vi "GEA3 Heat Pump ERD List.vi"(8 "error in (no error)":errorcluster, 11 "Enable Heat Pump List":bool) -> (0 "error out":errorcluster, 2 "Headers":string[](array[string]), 3 "Read ERD List":T1[](array[typedef]) {"ERD Number" format="%.0x"})   [LabVIEW 2020]
uses:
  type defs/ERD Read Data In.ctl
  type defs/Data Type.ctl
  <vilib>/Utility/error.llb/whitespace.ctl
  library/GEA2_Toolkit.lvlib
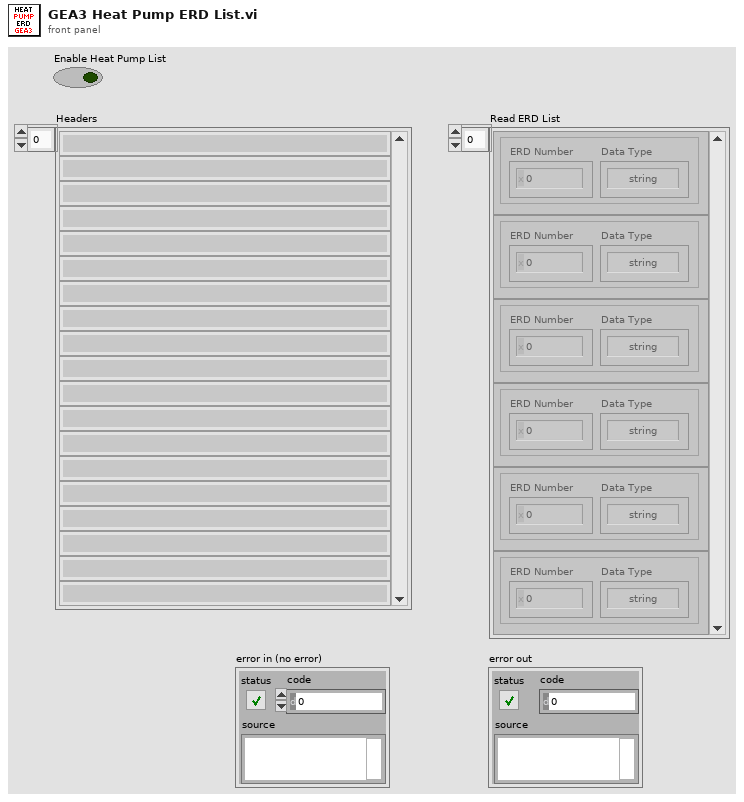
[diagram p1: front panel]
types:
  T1 = typedef "GEA2_Toolkit.lvlib/ERD Read Data In.ctl" = cluster{"ERD Number":u16, "Data Type":T2}
  T2 = typedef "GEA2_Toolkit.lvlib/Data Type.ctl" = enum16{"string", "boolean", "uint8_t", "uint16_t", "uint32_t", "uint64_t", "int8_t", "int16_t", "int32_t", "int64_t"}
  T3 = typedef "whitespace.ctl" = u16
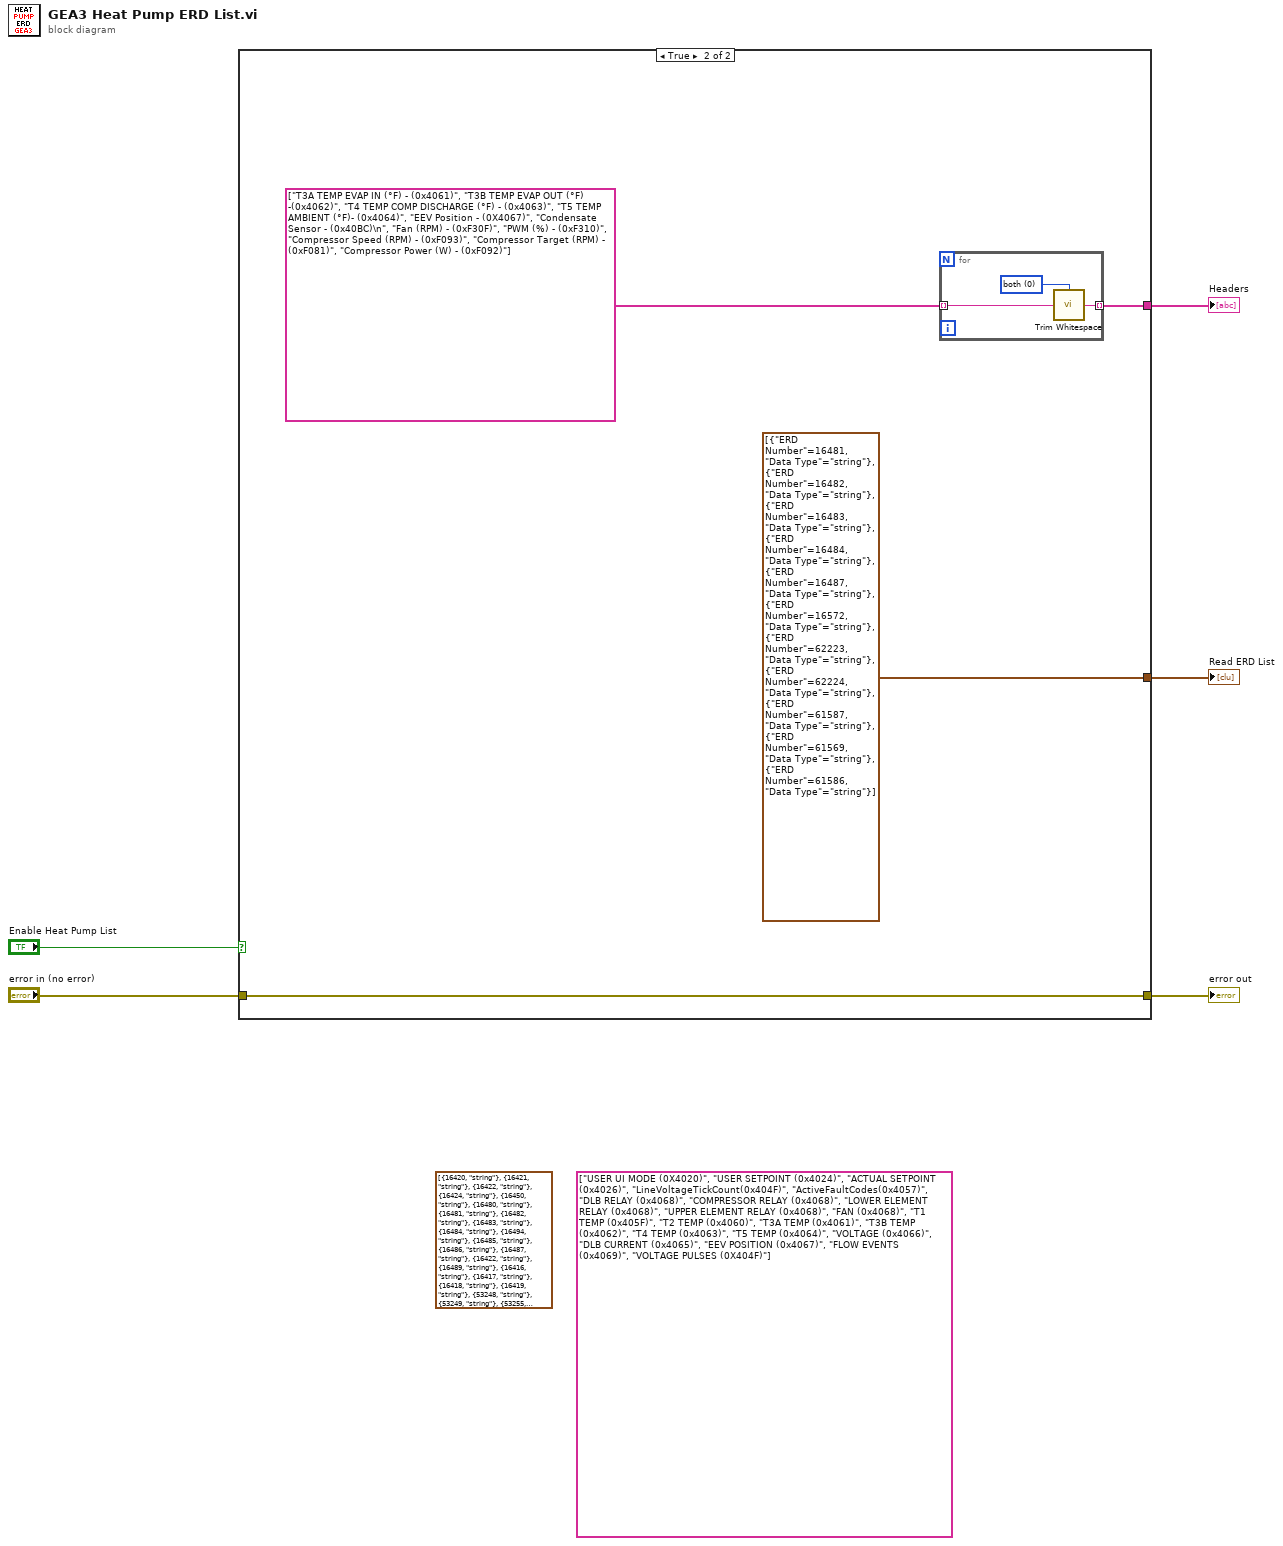
[diagram p0: block diagram]
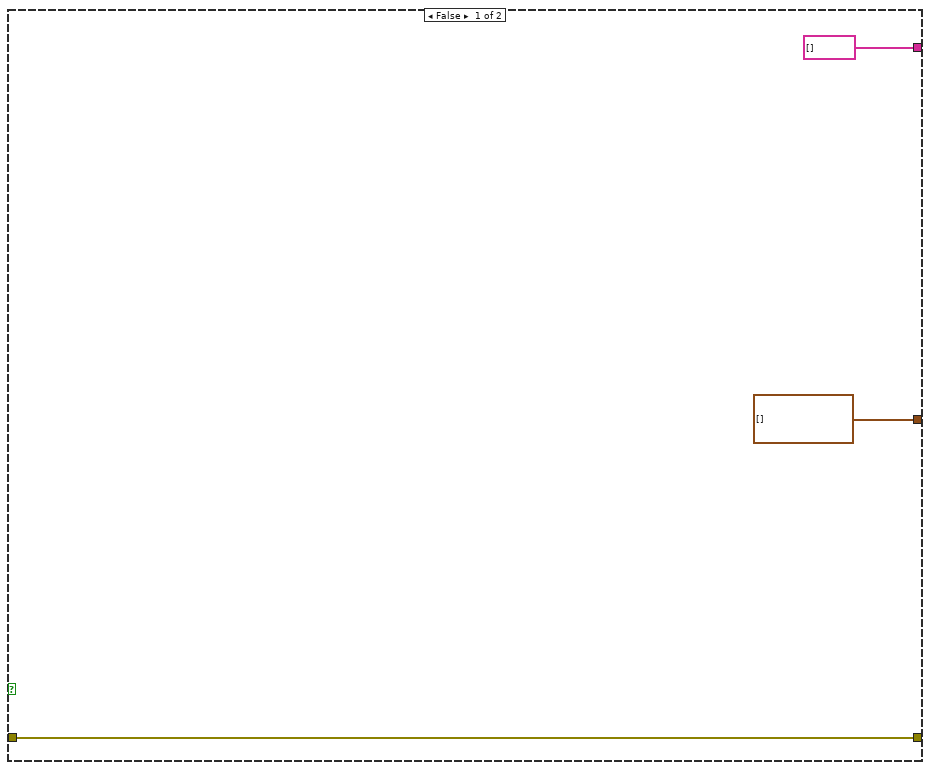
[diagram p2: hidden frame]
diagram:
  (unwired) T1[] [{"ERD Number"=16420, "Data Type"=enum."string"}, {"ERD Number"=16421, "Data Type"=enum."string"}, {"ERD Number"=16422, "Data Type"=enum."string"}, {"ERD Number"=16424, "Data Type"=enum."string"}, {"ERD Number"=16450, "Data Type"=enum."string"}, {"ERD Number"=16480, "Data Type"=enum."string"}, {"ERD Number"=16481, "Data Type"=enum."string"}, {"ERD Number"=16482, "Data Type"=enum."string"}, {"ERD Number"=16483, "Data Type"=enum."string"}, {"ERD Number"=16484, "Data Type"=enum."string"}, {"ERD Number"=16494, "Data Type"=enum."string"}, {"ERD Number"=16485, "Data Type"=enum."string"}, {"ERD Number"=16486, "Data Type"=enum."string"}, {"ERD Number"=16487, "Data Type"=enum."string"}, {"ERD Number"=16422, "Data Type"=enum."string"}, {"ERD Number"=16489, "Data Type"=enum."string"}, {"ERD Number"=16416, "Data Type"=enum."string"}, {"ERD Number"=16417, "Data Type"=enum."string"}, {"ERD Number"=16418, "Data Type"=enum."string"}, {"ERD Number"=16419, "Data Type"=enum."string"}, {"ERD Number"=53248, "Data Type"=enum."string"}, {"ERD Number"=53249, "Data Type"=enum."string"}, {"ERD Number"=53255, "Data Type"=enum."string"}, {"ERD Number"=53256, "Data Type"=enum."string"}, {"ERD Number"=16453, "Data Type"=enum."string"}, {"ERD Number"=16497, "Data Type"=enum."string"}, {"ERD Number"=16488, "Data Type"=enum."string"}, {"ERD Number"=16491, "Data Type"=enum."string"}, {"ERD Number"=16492, "Data Type"=enum."string"}] ("Read ERD List")
  (unwired) string[] ["USER UI MODE (0X4020)", "USER SETPOINT (0x4024)", "ACTUAL SETPOINT (0x4026)", "LineVoltageTickCount(0x404F)", "ActiveFaultCodes(0x4057)", "DLB RELAY (0x4068)", "COMPRESSOR RELAY (0x4068)", "LOWER ELEMENT RELAY (0x4068)", "UPPER ELEMENT RELAY (0x4068)", "FAN (0x4068)", "T1 TEMP (0x405F)", "T2 TEMP (0x4060)", "T3A TEMP (0x4061)", "T3B TEMP (0x4062)", "T4 TEMP (0x4063)", "T5 TEMP (0x4064)", "VOLTAGE (0x4066)", "DLB CURRENT (0x4065)", "EEV POSITION (0x4067)", "FLOW EVENTS (0x4069)", "VOLTAGE PULSES (0X404F)"]
  n1 = case shown="True" "Enable Heat Pump List" {
    tunnel: [T1[] [] ("Read ERD List") T1[] [{"ERD Number"=16481, "Data Type"=enum."string"}, {"ERD Number"=16482, "Data Type"=enum."string"}, {"ERD Number"=16483, "Data Type"=enum."string"}, {"ERD Number"=16484, "Data Type"=enum."string"}, {"ERD Number"=16487, "Data Type"=enum."string"}, {"ERD Number"=16572, "Data Type"=enum."string"}, {"ERD Number"=62223, "Data Type"=enum."string"}, {"ERD Number"=62224, "Data Type"=enum."string"}, {"ERD Number"=61587, "Data Type"=enum."string"}, {"ERD Number"=61569, "Data Type"=enum."string"}, {"ERD Number"=61586, "Data Type"=enum."string"}] ("Read ERD List")] -> w5
    tunnel: "error in (no error)" -> [w8 w11]
    tunnel: [w8 w11] -> w3
    tunnel: [string[] [] ("array") w10] -> w1
    frame False {
    }
    frame True {
      n2 = for {
        tunnel: string[] ["T3A TEMP EVAP IN (°F) - (0x4061)", "T3B TEMP EVAP OUT (°F) -(0x4062)", "T4 TEMP COMP DISCHARGE (°F) - (0x4063)", "T5 TEMP AMBIENT (°F)- (0x4064)", "EEV Position - (0X4067)", "Condensate Sensor - (0x40BC)\n", "Fan (RPM) - (0xF30F)", "PWM (%) - (0xF310)", "Compressor Speed (RPM) - (0xF093)", "Compressor Target (RPM) - (0xF081)", "Compressor Power (W) - (0xF092)"] -> [w14] mode=indexing
        tunnel: [w13] -> w10 mode=indexing
        w15 = T3 0 items=["both", "start of string", "end of string"] ("location (both)")
        n3 = call <vilib>:"Trim Whitespace.vi"("string"=w14, "location (both)"=w15) -> ("trimmed string"=w13:string)
      }
    }
  }
  "Read ERD List" <- w5
  "Headers" <- w1
  "error out" <- w3
